vi "Digital multimeter.vi"() -> ()   [LabVIEW 2021]
uses:
  Main states enum-digital.ctl
  Globals/Global message.vi
  Globals/CH1.vi
panel:
  in  "Hold":bool
  in  "Knob":u32(knob)=3 step=1 scale=0.0..10.0
  in  "Stop Button":bool
  out "Indicator":dbl format="%_3g"
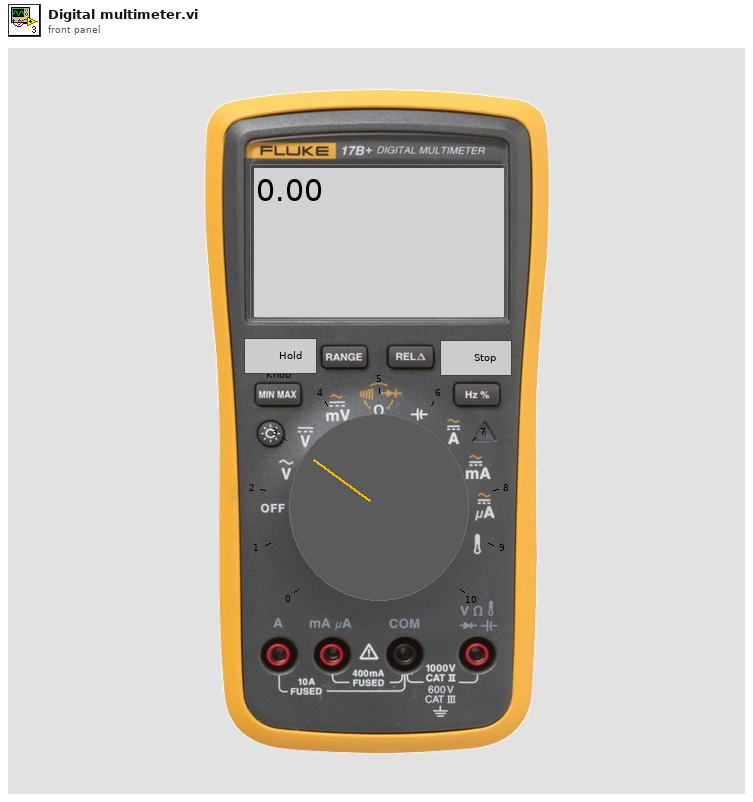
[diagram p1: front panel]
types:
  T1 = cluster{"Voltage":dbl, "Current":dbl, "Message":string}
  T2 = typedef "Main states enum-digital.ctl" = enum16{"Initialize", "Update", "Stop"}
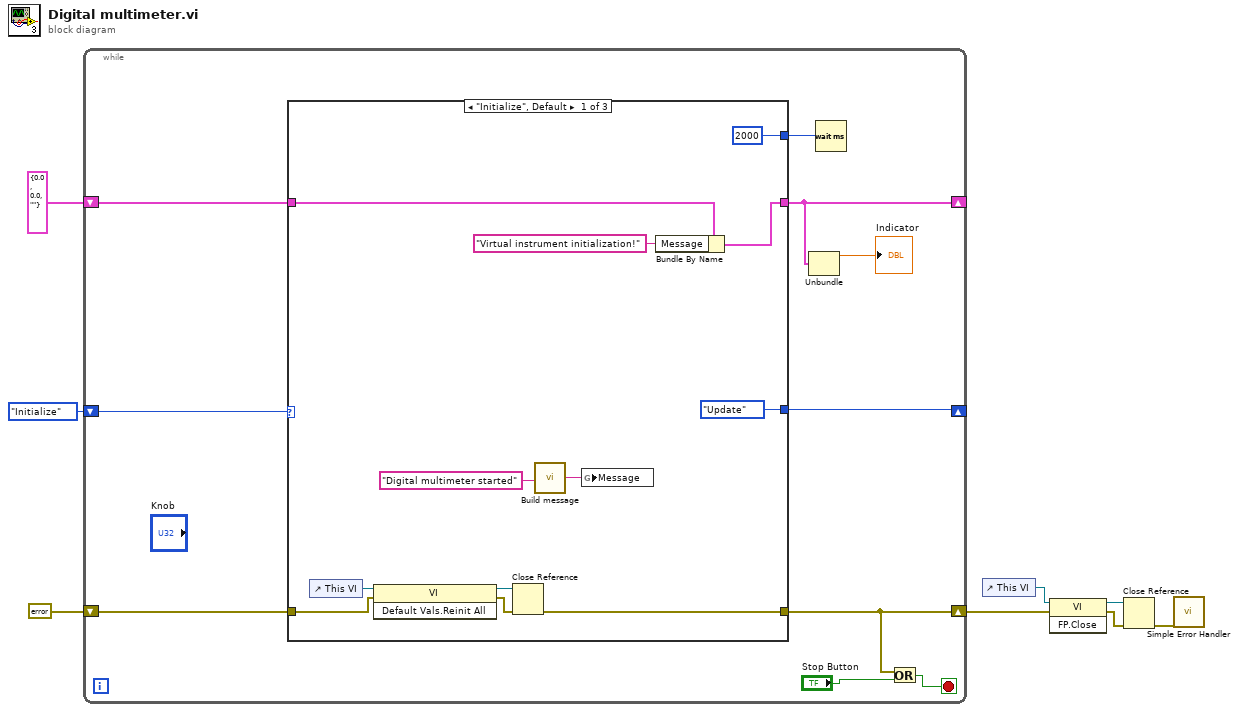
[diagram p0: block diagram]
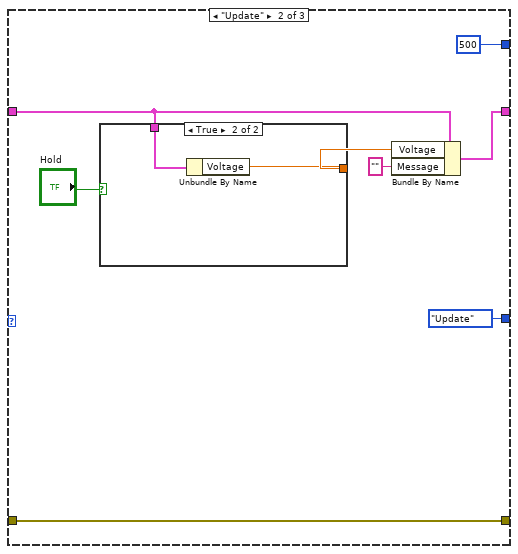
[diagram p2: hidden frame]
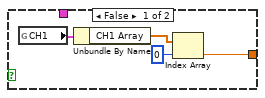
[diagram p3: hidden frame]
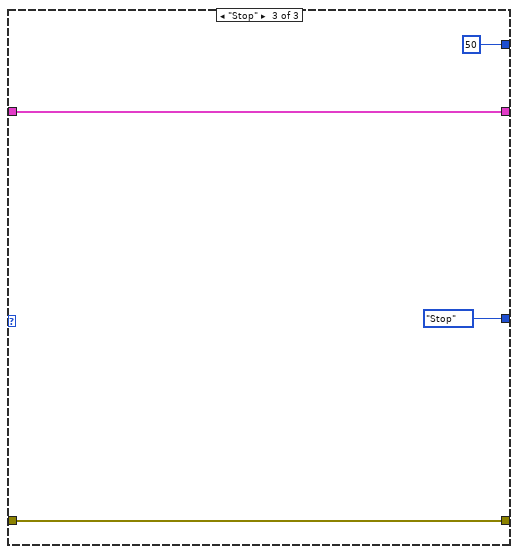
[diagram p4: hidden frame]
diagram:
  n1 = while {
    shift-right: [w16] -> w6
    shift-left: errorcluster {"status"=FALSE, "code"=0, "source"=""} ("error constant") -> [w18]
    shift-right: [w12] -> _
    shift-left: T1 {"Voltage"=0.0, "Current"=0.0, "Message"=""} -> [w15]
    shift-right: [w13] -> _
    shift-left: Main_states_enum-digital."Initialize" ("Enum") -> [w14]
    stop <- w17 stop-if-true
    n2 = case shown="\"Initialize\", Default" w14 {
      tunnel: w18 -> [w27 w38 w47]
      tunnel: [w21 w38 w47] -> w16
      tunnel: w15 -> [w23 w31 w45]
      tunnel: [w22 w36 w45] -> w12
      tunnel: [Main_states_enum-digital."Update" ("Enum") Main_states_enum-digital."Update" ("Enum") Main_states_enum-digital."Stop" ("Enum")] -> w13
      tunnel: [u32 2000 ("milliseconds to wait") u32 500 ("milliseconds to wait") u32 50 ("milliseconds to wait")] -> w11
      frame "Initialize", Default {
        n3 = control-ref of="This VI"() -> (w30:refnum<vi>)
        n4 = invoke class="VI" method="Default Vals.Reinit All"(reference=w30, error in=w27) -> (reference out=w29:refnum<vi>, error out=w28:errorcluster)  [unwired: 1 in, 1 out]
        n5 = Close Reference(reference=w29, error in (no error)=w28) -> (error out=w21:errorcluster)
        n6 = call "Build message.vi"("Input string"="Digital multimeter started") -> ("Output string"=w19:string)
        n7 = global write "Global message.vi" "Message"(w19) -> ()
        n8 = Bundle By Name(cluster=w23, "Message"="Virtual instrument initialization!") -> (w22:T1)
      }
      frame "Update" {
        n9 = case shown="True" "Hold" {
          tunnel: [w39 w43] -> w33
          tunnel: w31 -> [_ w44]
          frame False {
            n10 = global read "CH1.vi" "CH1"() -> (w42:cluster{"CH1 Array":dbl[], "CH1 Message":string})
            n11 = Unbundle By Name(w42) -> ("CH1 Array"=w41:dbl[])
            n12 = Index Array(array=w41, index=0) -> (element=w39:dbl)
          }
          frame True {
            n13 = Unbundle By Name(w44) -> ("Voltage"=w43:dbl)
          }
        }
        n14 = Bundle By Name(cluster=w31, "Voltage"=w33, "Message"="") -> (w36:T1)
      }
      frame "Stop" {
      }
    }
    n15 = Unbundle(w12) -> ("Voltage"=→"Indicator":dbl)  [unwired: 2 out]
    n16 = Wait (ms)(milliseconds to wait=w11) -> ()  [unwired: 1 out]
    n17 = Or(x=w16, y="Stop Button") -> (x .or. y?=w17:bool)
  }
  n18 = control-ref of="This VI"() -> (w3:refnum<vi>)
  n19 = invoke class="VI" method="FP.Close"(reference=w3, error in=w6) -> (reference out=w1:refnum<vi>, error out=w2:errorcluster)  [unwired: 1 in, 1 out]
  n20 = Close Reference(reference=w1, error in (no error)=w2) -> (error out=w5:errorcluster)
  n21 = call <vilib>:"Simple Error Handler.vi"("error in (no error)"=w5) -> ()  [unwired: 4 in, 5 out]
